vi "findKey.vi"(8 "Body In":string, 9 "offset (0)":i32, 10 "Cutoff Text":string="Back to Top", 11 "Key":string=") Summary: ") -> (2 "Val2":string, 3 "Val out":string)   [LabVIEW 2013]
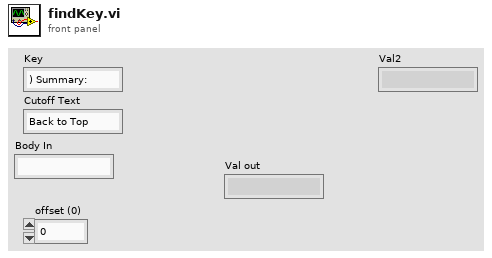
[diagram p1: front panel]
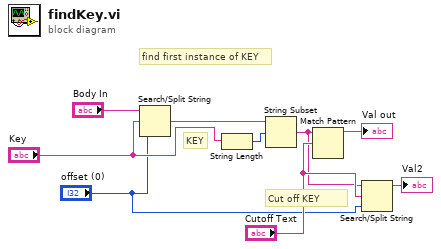
[diagram p0: block diagram]
diagram:
  # "Cut off KEY"
  # "KEY"
  # "find first instance of KEY"
  n1 = Search/Split String(string="Body In", search string/char (-)="Key", offset (0)="offset (0)") -> (match + rest of string=w8:string)  [unwired: 2 out]
  n2 = String Length(string="Key") -> (length=w9:i32)
  n3 = String Subset(string=w8, offset (0)=w9) -> (substring=w3:string)  [unwired: 1 in]
  n4 = Match Pattern(string=w3, regular expression="Cutoff Text") -> (before substring=→"Val out":string)  [unwired: 1 in, 3 out]
  n5 = Search/Split String(string=w3, search string/char (-)="Cutoff Text", offset (0)="offset (0)") -> (substring before match=→"Val2":string)  [unwired: 2 out]
